vi "ColourSelector.vi"(8 "error in (no error)":errorcluster, 11 "Bool Refnum":refnum<vi>) -> (0 "error out":errorcluster={"status"=TRUE, "code"=1055, "source"="Property Node in ColourSelector.vi"})   [LabVIEW 2014]
panel:
  out "Example":bool[][](array[boolean])=[[FALSE, FALSE, FALSE, FALSE, FALSE, FALSE, FALSE, FALSE, FALSE, FALSE, FALSE, FALSE, FALSE, FALSE, FALSE, FALSE, FALSE], [FALSE, TRUE, TRUE, FALSE, FALSE, TRUE, TRUE, TRUE, TRUE, TRUE, TRUE, TRUE, FALSE, FALSE, TRUE, TRUE, FALSE], [FALSE, TRUE, FALSE, FALSE, TRUE, TRUE, TRUE, TRUE, TRUE, TRUE, TRUE, TRUE, TRUE, FALSE, FALSE, TRUE, FALSE], [FALSE, FALSE, FALSE, TRUE, TRUE, FALSE, FALSE, FALSE, FALSE, FALSE, FALSE, FALSE, TRUE, TRUE, FALSE, FALSE, FALSE], [FALSE, FALSE, TRUE, TRUE, FALSE, FALSE, TRUE, FALSE, FALSE, FALSE, TRUE, FALSE, FALSE, TRUE, TRUE, FALSE, FALSE], [FALSE, TRUE, TRUE, FALSE, FALSE, TRUE, TRUE, TRUE, FALSE, TRUE, TRUE, TRUE, FALSE, FALSE, TRUE, TRUE, FALSE], [FALSE, TRUE, TRUE, FALSE, TRUE, TRUE, TRUE, TRUE, FALSE, TRUE, TRUE, TRUE, TRUE, FALSE, TRUE, TRUE, FALSE], [FALSE, TRUE, TRUE, FALSE, TRUE, TRUE, TRUE, TRUE, FALSE, TRUE, TRUE, TRUE, TRUE, FALSE, TRUE, TRUE, FALSE], [FALSE, TRUE, TRUE, FALSE, FALSE, TRUE, TRUE, FALSE, FALSE, FALSE, TRUE, TRUE, FALSE, FALSE, TRUE, TRUE, FALSE], [FALSE, TRUE, TRUE, FALSE, FALSE, FALSE, FALSE, FALSE, FALSE, FALSE, FALSE, FALSE, FALSE, FALSE, TRUE, TRUE, FALSE], [FALSE, TRUE, TRUE, FALSE, TRUE, TRUE, FALSE, FALSE, FALSE, FALSE, FALSE, TRUE, TRUE, FALSE, TRUE, TRUE, FALSE], [FALSE, TRUE, TRUE, FALSE, FALSE, TRUE, TRUE, TRUE, TRUE, TRUE, TRUE, TRUE, FALSE, FALSE, TRUE, TRUE, FALSE], [FALSE, FALSE, TRUE, TRUE, FALSE, FALSE, TRUE, TRUE, TRUE, TRUE, TRUE, FALSE, FALSE, TRUE, TRUE, FALSE, FALSE], [FALSE, FALSE, FALSE, TRUE, TRUE, FALSE, FALSE, FALSE, FALSE, FALSE, FALSE, FALSE, TRUE, TRUE, FALSE, FALSE, FALSE], [FALSE, FALSE, FALSE, FALSE, TRUE, TRUE, TRUE, TRUE, TRUE, TRUE, TRUE, TRUE, TRUE, FALSE, FALSE, FALSE, FALSE], [FALSE, FALSE, FALSE, FALSE, FALSE, TRUE, TRUE, TRUE, TRUE, TRUE, TRUE, TRUE, FALSE, FALSE, FALSE, FALSE, FALSE]]
  in  "Select":bool
  in  "LED Colour (False)":u32(colorbox)=3997440
  in  "LED Colour (True)":u32(colorbox)=940800
  # "OK, before we get started...\nPlease select the foreground and \nbackground colours for the Dot Matrix"
  # "Example \nDot Matrix"
  # "Foreground"
  # "Background"
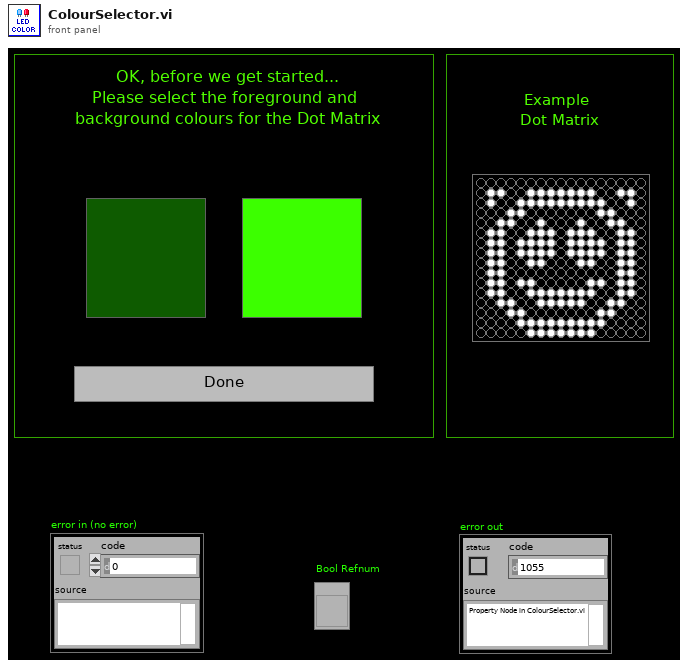
[diagram p1: front panel]
types:
  T1 = cluster{"LED Colour (True)":u32, "LED Colour (True) 2":u32}[]
  T2 = cluster{"LED Colour (False)":u32, "LED Colour (False)":u32}
  T3 = cluster{"LED Colour (True)":u32, "LED Colour (True)":u32}
  T4 = cluster{"LED Colour (False)":u32, "LED Colour (False)":u32}[]
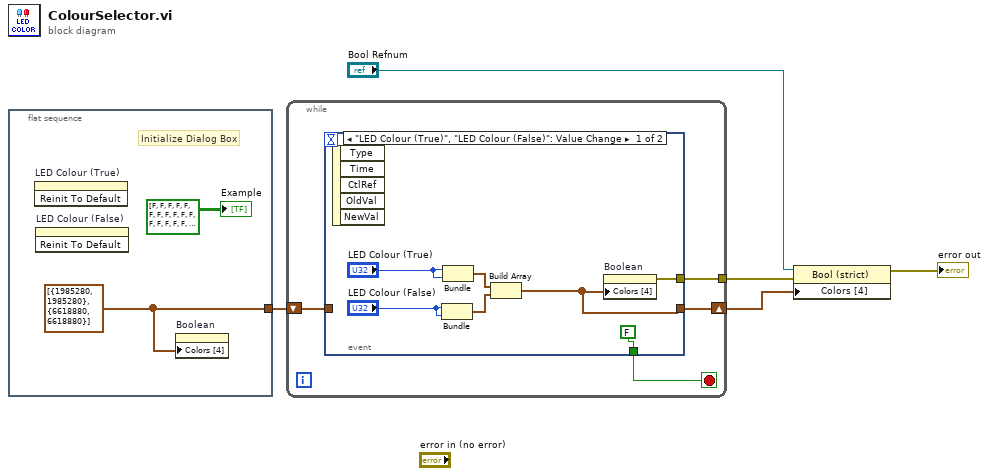
[diagram p0: block diagram]
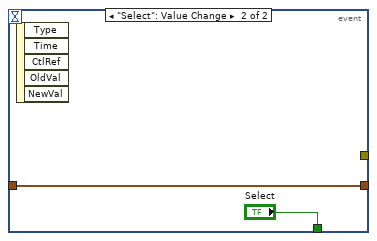
[diagram p2: hidden frame]
diagram:
  n1 = flat-sequence {
    tunnel: [w6] -> w1
    frame #0 {
      w6 = T1 [{"LED Colour (True)"=1985280, "LED Colour (True) 2"=1985280}, {"LED Colour (True)"=6618880, "LED Colour (True) 2"=6618880}]
      # "Initialize Dialog Box"
      n2 = invoke on="LED Colour (True)" class="ColBox" method="Reinit To Default"() -> ()  [unwired: 3 in, 3 out]
      n3 = invoke on="LED Colour (False)" class="ColBox" method="Reinit To Default"() -> ()  [unwired: 3 in, 3 out]
      n4 = property on="Boolean" class="Bool (strict)"("Colors [4]"=w6) -> ()  [unwired: 2 in, 2 out]
      "Example" <- bool[][] [[FALSE, FALSE, FALSE, FALSE, FALSE, FALSE, FALSE, FALSE, FALSE, FALSE, FALSE, FALSE, FALSE, FALSE, FALSE, FALSE, FALSE], [FALSE, TRUE, TRUE, FALSE, FALSE, TRUE, TRUE, TRUE, TRUE, TRUE, TRUE, TRUE, FALSE, FALSE, TRUE, TRUE, FALSE], [FALSE, TRUE, FALSE, FALSE, TRUE, TRUE, TRUE, TRUE, TRUE, TRUE, TRUE, TRUE, TRUE, FALSE, FALSE, TRUE, FALSE], [FALSE, FALSE, FALSE, TRUE, TRUE, FALSE, FALSE, FALSE, FALSE, FALSE, FALSE, FALSE, TRUE, TRUE, FALSE, FALSE, FALSE], [FALSE, FALSE, TRUE, TRUE, FALSE, FALSE, TRUE, FALSE, FALSE, FALSE, TRUE, FALSE, FALSE, TRUE, TRUE, FALSE, FALSE], [FALSE, TRUE, TRUE, FALSE, FALSE, TRUE, TRUE, TRUE, FALSE, TRUE, TRUE, TRUE, FALSE, FALSE, TRUE, TRUE, FALSE], [FALSE, TRUE, TRUE, FALSE, TRUE, TRUE, TRUE, TRUE, FALSE, TRUE, TRUE, TRUE, TRUE, FALSE, TRUE, TRUE, FALSE], [FALSE, TRUE, TRUE, FALSE, TRUE, TRUE, TRUE, TRUE, FALSE, TRUE, TRUE, TRUE, TRUE, FALSE, TRUE, TRUE, FALSE], [FALSE, TRUE, TRUE, FALSE, FALSE, TRUE, TRUE, FALSE, FALSE, FALSE, TRUE, TRUE, FALSE, FALSE, TRUE, TRUE, FALSE], [FALSE, TRUE, TRUE, FALSE, FALSE, FALSE, FALSE, FALSE, FALSE, FALSE, FALSE, FALSE, FALSE, FALSE, TRUE, TRUE, FALSE], [FALSE, TRUE, TRUE, FALSE, TRUE, TRUE, FALSE, FALSE, FALSE, FALSE, FALSE, TRUE, TRUE, FALSE, TRUE, TRUE, FALSE], [FALSE, TRUE, TRUE, FALSE, FALSE, TRUE, TRUE, TRUE, TRUE, TRUE, TRUE, TRUE, FALSE, FALSE, TRUE, TRUE, FALSE], [FALSE, FALSE, TRUE, TRUE, FALSE, FALSE, TRUE, TRUE, TRUE, TRUE, TRUE, FALSE, FALSE, TRUE, TRUE, FALSE, FALSE], [FALSE, FALSE, FALSE, TRUE, TRUE, FALSE, FALSE, FALSE, FALSE, FALSE, FALSE, FALSE, TRUE, TRUE, FALSE, FALSE, FALSE], [FALSE, FALSE, FALSE, FALSE, TRUE, TRUE, TRUE, TRUE, TRUE, TRUE, TRUE, TRUE, TRUE, FALSE, FALSE, FALSE, FALSE], [FALSE, FALSE, FALSE, FALSE, FALSE, TRUE, TRUE, TRUE, TRUE, TRUE, TRUE, TRUE, FALSE, FALSE, FALSE, FALSE, FALSE]] ("Example")
    }
  }
  n5 = while {
    tunnel: [w11] -> w3
    shift-right: [w9] -> w2
    shift-left: w1 -> [w8]
    stop <- w10 stop-if-true
    n6 = event shown="[0] \"LED Colour (True)\", \"LED Colour (False)\": Value Change" {
      selector: _ -> [_ _]
      dyn-events: _ -> [_ _]
      timeout: _ -> [_ _]
      tunnel: [w14 _] -> w11
      tunnel: [FALSE ("Select") "Select"] -> w10
      tunnel: [w12 w19] -> w9
      tunnel: w8 -> [_ w19]
      event "LED Colour (True)", "LED Colour (False)": Value Change {
        n7 = event-data() -> ()  [unwired: 1 in, 5 out]
        n8 = Bundle("LED Colour (False)"="LED Colour (False)", "LED Colour (False)"="LED Colour (False)") -> (w15:T2)  [unwired: 1 in]
        n9 = Bundle("LED Colour (True)"="LED Colour (True)", "LED Colour (True)"="LED Colour (True)") -> (w16:T3)  [unwired: 1 in]
        n10 = Build Array(w16, w15) -> (w12:T4)
        n11 = property on="Boolean" class="Bool (strict)"("Colors [4]"=w12) -> (error out=w14:errorcluster)  [unwired: 2 in, 1 out]
      }
      event "Select": Value Change {
        n12 = event-data() -> ()  [unwired: 1 in, 5 out]
      }
    }
  }
  n13 = property on="Property Node" class="Bool (strict)"(reference="Bool Refnum", error in=w3, "Colors [4]"=w2) -> (error out=→"error out":errorcluster)  [unwired: 1 out]
